vi "PI MVR.vi"(8 "error in (no error)":errorcluster, 10 "String":string, 11 "PI ID in":i32) -> (0 "error out":errorcluster, 2 "szCommand":string, 3 "PI ID out":i32)   [LabVIEW 2020]
uses:
  Low Level/GCSTranslator.dll
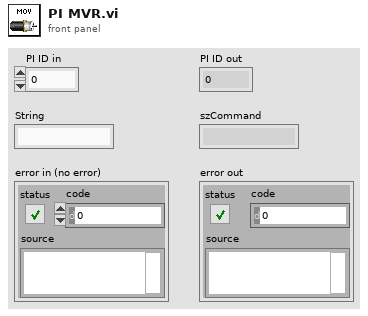
[diagram p1: front panel]
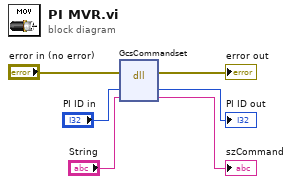
[diagram p0: block diagram]
diagram:
  n1 = dll-call lib="D:/software/TweezerTron Project/Instruments/Physik Instrumente/SDK/GCS_LabVIEW_digital/Low Level/GCSTranslator.dll" fn="GcsCommandset" label="Send Command"(error in="error in (no error)", "ID"="PI ID in", "szCommand"="String") -> (error out=→"error out":errorcluster, "ID"=→"PI ID out":i32, "szCommand"=→"szCommand":string)  [unwired: 2 in, 2 out]
